vi "ProcessSensorData.vi"(8 "error in (no error)":errorcluster, 11 "CorrFactor":refnum<class "CorrFactor.lvclass">) -> (0 "error out":errorcluster, 2 "TimedOout":bool, 3 "CorrFactor":refnum<class "CorrFactor.lvclass">)   [LabVIEW 2018, in "AnalysisPlugins.lvlib" / "CorrFactor.lvclass"]
uses:
  CorrFactor.lvclass
  C:/projects/ICDAS/NistPluggableModules/Analysis/AnalysisPlugins/AnalysisPluginBaseClass/AnalysisPluginsBase.lvclass
  AnalysisPluginBaseClass/AnalysisPluginsBase.lvclass/AnalysisPluginsBase.ctl
  PmuAnalysisClass/Typedefs/PmuData.ctl
  AnalysisPluginBaseClass/Accessors/Write AnalysisTime.vi
  AnalysisPluginBaseClass/Accessors/Read SensorQue.vi
  PmuAnalysisClass/PmuAnalysis.lvclass
panel:
  out "TimeStamp":timestamp
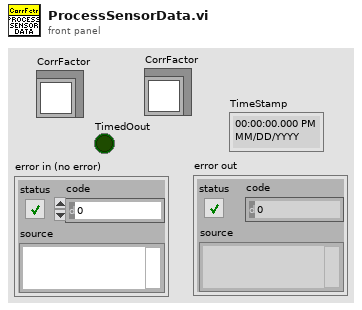
[diagram p1: front panel]
types:
  T1 = typedef "AnalysisPlugins.lvlib/PmuAnalysis.lvclass/PmuData.ctl" = cluster{"Timestamp":dbl, "Synx":cdb[], "Freq":dbl, "ROCOF":dbl, "ID":i16}
  T2 = typedef "SensorQueue.ctl" = refnum<queue>
  T3 = typedef "AnalysisPlugins.lvlib/AnalysisPluginsBase.lvclass/clSensorData.ctl" = cluster{"SensorType":string, "SensorData":variant, "TimeStamp":timestamp}
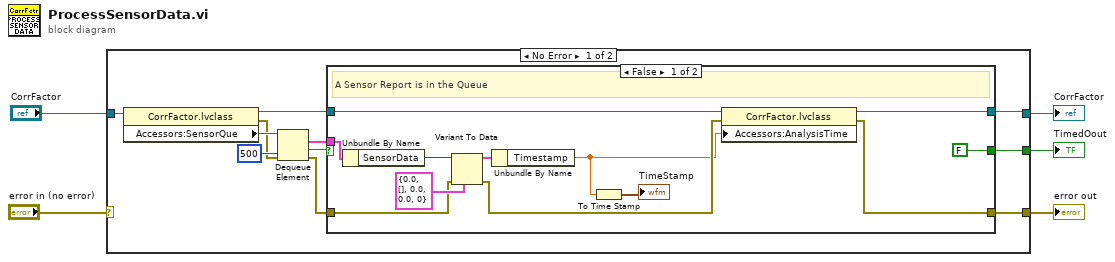
[diagram p0: block diagram]
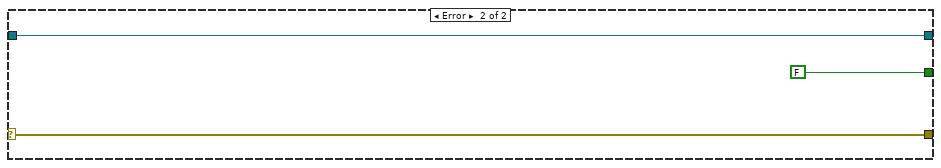
[diagram p3: hidden frame]
diagram:
  n1 = case shown="No Error" "error in (no error)" {
    selector: "error in (no error)" -> [_ w34]
    tunnel: [w10 w34] -> w4
    tunnel: "CorrFactor" -> [w16 w33]
    tunnel: [w7 w33] -> w2
    tunnel: [w11 FALSE] -> w1
    frame No Error {
      n2 = property class="CorrFactor.lvclass"(reference=w16) -> (reference out=w8:refnum<class "CorrFactor.lvclass">, error out=w13:errorcluster, "Accessors:SensorQue"=w15:T2)  [unwired: 1 in]
      n3 = Dequeue Element(queue=w15, timeout in ms (-1)=500, error in (no error)=w13) -> (element=w9:T3, timed out?=w12:bool, error out=w6:errorcluster)  [unwired: 1 out]
      n4 = case shown="False" w12 {
        selector: w12 -> [_ w31]
        tunnel: [FALSE w31] -> w11
        tunnel: w6 -> [w20 w30]
        tunnel: [w24 w30] -> w10
        tunnel: w9 -> [w28 _]
        tunnel: w8 -> [w27 w29]
        tunnel: [w25 w29] -> w7
        frame False {
          # "A Sensor Report is in the Queue"
          n5 = Unbundle By Name(w28) -> ("SensorData"=w23:variant)
          n6 = Variant To Data(error in=w20, type=T1 {"Timestamp"=0.0, "Synx"=[], "Freq"=0.0, "ROCOF"=0.0, "ID"=0} ("PmuReport"), Variant=w23) -> (data=w19:T1, error out=w21:errorcluster)
          n7 = Unbundle By Name(w19) -> ("Timestamp"=w17:dbl)
          n8 = To Time Stamp(1:w17) -> (0:→"TimeStamp":timestamp)
          n9 = property class="CorrFactor.lvclass"(reference=w27, error in=w21, "Accessors:AnalysisTime"=w17) -> (reference out=w25:refnum<class "CorrFactor.lvclass">, error out=w24:errorcluster)
        }
        frame True {
          # "Queue Timed out, allow the loop to run to check for stop state"
        }
      }
    }
    frame Error {
    }
  }
  "CorrFactor" <- w2
  "error out" <- w4
  "TimedOout" <- w1
